vi "COLL_Write_Config.vi"(4 "error in (no error)":errorcluster, 7 "Config Refnum":T1) -> (0 "error out":errorcluster, 3 "refnum out":T1)   [LabVIEW 2015]
uses:
  <vilib>/Utility/config.llb/Config Data RefNum.ctl
  <vilib>/Utility/config.llb/NI_LVConfig.lvlib
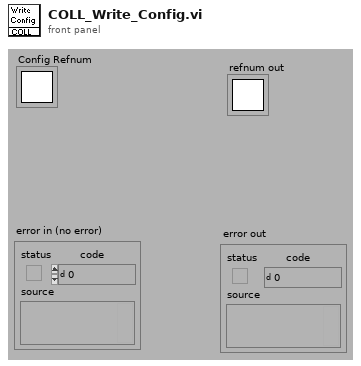
[diagram p1: front panel]
types:
  T1 = typedef "NI_LVConfig.lvlib/Config Data RefNum.ctl" = refnum<k1>
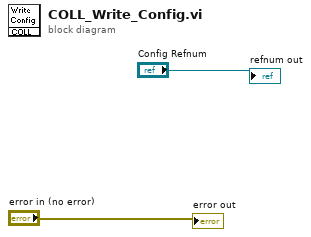
[diagram p0: block diagram]
diagram:
  "error out" <- "error in (no error)"
  "refnum out" <- "Config Refnum"
